vi "Add.vi"(8 "error in (no error)":errorcluster, 9 "LabVIEW Object":refnum<class>, 10 "key":string, 11 "Object Dictionary in (new)":refnum<class "objdict.lvclass">) -> (0 "error out":errorcluster, 3 "Object Dictionary out":refnum<class "objdict.lvclass">)   [LabVIEW 2015, in "objdict.lvclass"]
doc: "Adds an object to the dictionary.\n\n<b>This VI is fast but unsafe:</b> if the specified key is already in use by another object, the Data Value Reference holding that object will be lost. This could cause a memory leak. An error is thrown by this VI if that happens. If safe behavior is required, use <b>Add or Replace.vi</b>, instead."
uses:
  objdict.lvclass
  objdict.lvclass/objdict.ctl
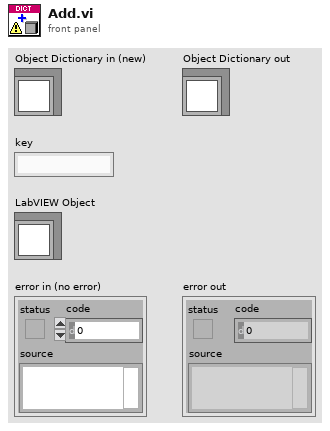
[diagram p1: front panel]
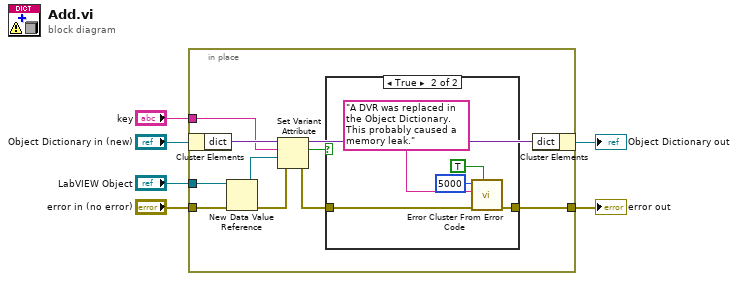
[diagram p0: block diagram]
diagram:
  n1 = in-place {
    in-place-border: [w8] -> w4
    in-place-border: "error in (no error)" -> [w16]
    in-place-border: "LabVIEW Object" -> [w11]
    in-place-border: "key" -> [w10]
    n2 = in-place-cluster #1("Object Dictionary in (new)") -> ("dict"=w14:variant)
    n3 = New Data Value Reference(data value=w11, error in=w16) -> (data value reference=w9:refnum<data-value>, error out=w12:errorcluster)
    n4 = Set Variant Attribute(Variant=w14, name=w10, value=w9, error in=w12) -> (Variant out=w13:variant, replaced=w7:bool, error out=w15:errorcluster)
    n5 = case shown="True" w7 {
      tunnel: w15 -> [w17 w22]
      tunnel: [w17 w21] -> w8
      frame False {
      }
      frame True {
        n6 = call <vilib>:"Error Cluster From Error Code.vi"("show call chain? (False)"=TRUE, "error in (no error)"=w22, "error message (\"\")"="A DVR was replaced in the Object Dictionary. This probably caused a memory leak.", "error code (0)"=5000) -> ("error out"=w21:errorcluster)  [unwired: 5 in]
      }
    }
    n7 = in-place-cluster #1("dict"=w13) -> (→"Object Dictionary out":refnum<class "objdict.lvclass">)
  }
  "error out" <- w4
